vi "Initialize Current Interval Indicator.vi"(3 "Protocol":T1[](array[typedef])) -> (1 "Current Interval Indicator":bool[](array[boolean]))   [LabVIEW 2019]
uses:
  Controls/Protocol Interval.ctl
  Controls/Stim Interval Mode.ctl
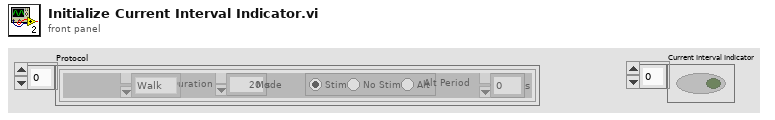
[diagram p1: front panel]
types:
  T1 = typedef "Protocol Interval.ctl" = cluster{"Interval Type":enum16{"Walk", "Rest"}, "Duration":dbl[unit], " Mode":T2, "Alt Period":dbl[unit]}
  T2 = typedef "Stim Interval Mode.ctl" = enum32{"Stim", "No Stim", "Alternating"}
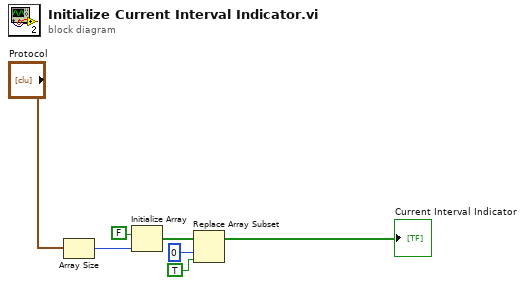
[diagram p0: block diagram]
diagram:
  n1 = Array Size(array="Protocol") -> (size(s)=w1:i32)
  n2 = Initialize Array(FALSE, w1) -> (w3:bool[])
  n3 = Replace Array Subset(array=w3, new element=TRUE ("new element/subarray"), index=0) -> (→"Current Interval Indicator":bool[])
